vi "Initialize APSVG.vi"(11 "MW generator constants":T1={"Lower limit [GHz]"=8.0, "Upper limit [GHz]"=20.0, "Device name"="VDIYT7", "Connection"="", "Description"="VDI Tracking", "Connected"=FALSE}) -> (0 "error out":errorcluster, 3 "MW generator constants out":T1={"Lower limit [GHz]"=8.0, "Upper limit [GHz]"=20.0, "Device name"="VDIYT7", "Connection"="", "Description"="VDI Tracking", "Connected"=FALSE})   [LabVIEW 2024, in "THz source modeule.lvlib"]
uses:
  THz source modeule.lvlib
  ctl/THz MW generator constants.ctl
  <vilib>/Utility/error.llb/Trim Whitespace One-Sided.vi
panel:
  out "FW version":string
  out "Serial number":string
  out "Company":string
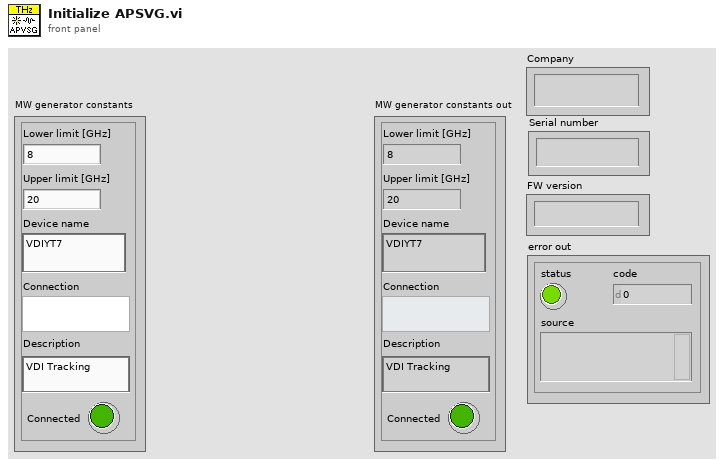
[diagram p1: front panel]
types:
  T1 = typedef "THz source modeule.lvlib/THz MW generator constants.ctl" = cluster{"Lower limit [GHz]":dbl, "Upper limit [GHz]":dbl, "Device name":string, "Connection":string, "Description":string, "Connected":bool}
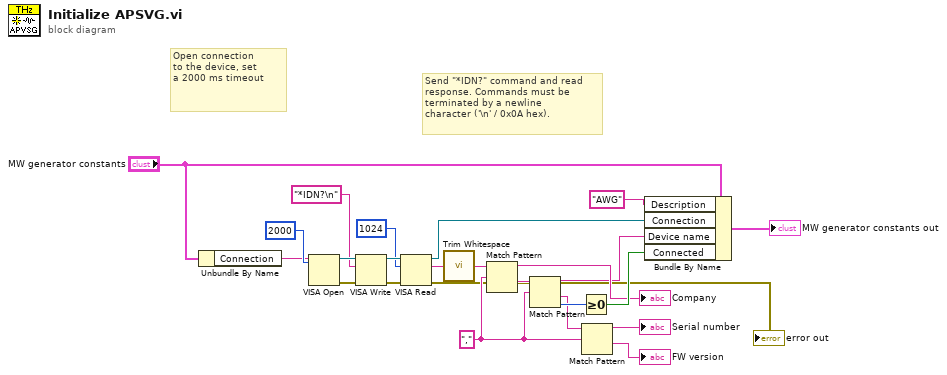
[diagram p0: block diagram]
diagram:
  w8 = "," ("regular expression")
  # "Send \"*IDN?\" command and read\nresponse. Commands must be\nterminated by a newline\ncharacter ('\\n' / 0x0A hex)."
  # "Open connection\nto the device, set\na 2000 ms timeout"
  n1 = Unbundle By Name("MW generator constants") -> ("Connection"=w15:string)
  n2 = VISA Open(timeout (0)=2000, VISA resource name=w15) -> (VISA resource name=w23:refnum<visa-resource-name>, error out=w22:errorcluster)  [unwired: 2 in, 1 out]
  n3 = VISA Write(VISA resource name=w23, write buffer="*IDN?\n", error in (no error)=w22) -> (VISA resource name out=w19:refnum<visa-resource-name>, error out=w20:errorcluster)  [unwired: 1 out]
  n4 = VISA Read(VISA resource name=w19, byte count=u32 1024, error in (no error)=w20) -> (VISA resource name out=w3:refnum<visa-resource-name>, read buffer=w24:string, error out=→"error out":errorcluster)  [unwired: 1 out]
  n5 = call <vilib>:"Trim Whitespace.vi"("string"=w24) -> ("trimmed string"=w10:string)  [unwired: 1 in]
  n6 = Match Pattern(string=w10, regular expression=w8) -> (before substring=→"Company":string, after substring=w16:string)  [unwired: 1 in, 2 out]
  n7 = Match Pattern(string=w16, regular expression=w8) -> (before substring=w2:string, after substring=w9:string, offset past match=w12:i32)  [unwired: 1 in, 1 out]
  n8 = Greater Or Equal To 0?(x=w12) -> (x >= 0?=w11:bool)
  n9 = Match Pattern(string=w9, regular expression=w8) -> (before substring=→"Serial number":string, after substring=→"FW version":string)  [unwired: 1 in, 2 out]
  n10 = Bundle By Name(cluster="MW generator constants", "Description"="AWG", "Connection"=w3, "Device name"=w2, "Connected"=w11) -> (→"MW generator constants out":T1)
